vi "SetDLLPath.vi"(8 "error in (no error)":errorcluster, 11 "DLLPath":path) -> (0 "error out":errorcluster)   [LabVIEW 2019]
doc: "Sets DLL Path and provides error in/out so that a race condition due to unset DLL Path is avoided"
uses:
  <userlib>/TaikoLaser/PDLM_DllPath_global.vi
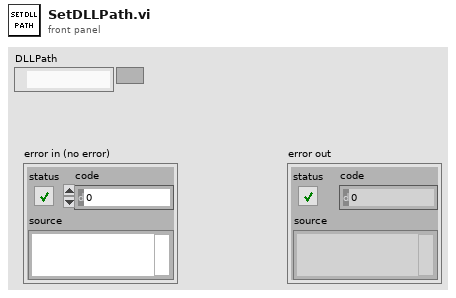
[diagram p1: front panel]
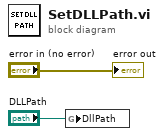
[diagram p0: block diagram]
diagram:
  n1 = global write "PDLM_DllPath_global.vi" "DllPath"("DLLPath") -> ()
  "error out" <- "error in (no error)"
